vi "Make Marker Delta.vi"(8 "error in (no error)":errorcluster {"code" format="%.0x"}, 9 "delta marker (Off)":bool, 11 "instrument handle":refnum<k15>) -> (0 "error out":errorcluster {"code" format="%.0x"}, 3 "instrument handle out":refnum<k15>)   [LabVIEW 2009, in "Keysight XSAn.lvlib"]
doc: "This VI specifies whether the active marker is a delta marker.\n\nSupported Models:M9290A, N8973B, N8974B, N8975B, N8976B, N9000A, N9000B, N9010A, N9010B, N9020A, N9020B, N9030A, N9030B, N9038A, N9040B, N9041B, SPN9003A, SPN9026A"
uses:
  <instrlib>/Keysight XSAn/Keysight XSAn.lvlib
  AgXSAn.dll
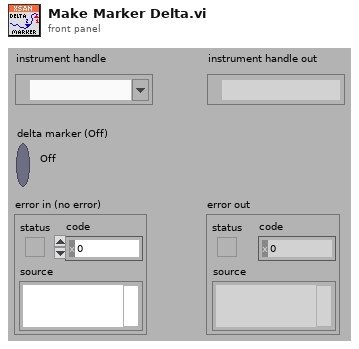
[diagram p1: front panel]
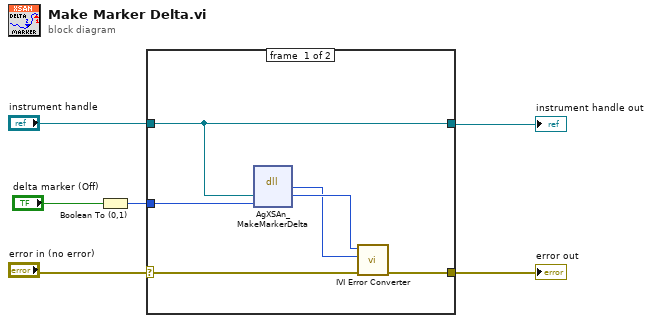
[diagram p0: block diagram]
diagram:
  n1 = Boolean To (0,1)(Boolean="delta marker (Off)") -> (0, 1=w1:i16)
  n2 = case shown="No Error" "error in (no error)" {
    selector: "error in (no error)" -> [w10 w14]
    tunnel: [w11 w14] -> w5
    tunnel: "instrument handle" -> [w8 w13]
    tunnel: [w8 w13] -> w3
    tunnel: w1 -> [w7 _]
    frame #0 {
      n3 = dll-call lib="AgXSAn**.dll" fn="AgXSAn_MakeMarkerDelta" ("LabVIEW:IviSpecAn_MakeMarkerDelta")("instrument handle"=w8, "delta marker"=w7) -> ("Status"=w9:i32, "instrument handle"=w12:u32)  [unwired: 4 in, 2 out]
      n4 = call <instrlib>:"IVI Error Converter.vi"("error in (no error)"=w10, "IVI error code (0)"=w9, "instrument handle"=w12) -> ("error out"=w11:errorcluster)  [unwired: 7 in, 1 out]
    }
    frame #1 {
    }
  }
  "error out" <- w5
  "instrument handle out" <- w3
